vi "测试类型1can应答.vi"(0 "输入切换ID":u8, 1 "输出切换ID":u8, 3 "匹配CANID":u32 format="%x") -> (8 "成功？":bool)   [LabVIEW 2010]
uses:
  全局量/全局_配置.vi
panel:
  out "开始时间":dbl format="%#.0f"
  out "接收数据":u8[](array[numeric])
  out "超时?":bool
  in  "Baudrate":u32(ring)=1000 caption="K" items=["10"=10, "20"=20, "50"=50, "100"=100, "125"=125, "250"=250, "500"=500, "800"=800, "250"=1000]
  in  "CANPort":u16
  in  "ReadTimeOut":u32=3000 caption="ms"
  in  "Synchronization":i32(ring)=1 items=["Synchronization"=1, "Asynchronization"=0]
  out "Error out":errorcluster {"code" format="%.0x"}
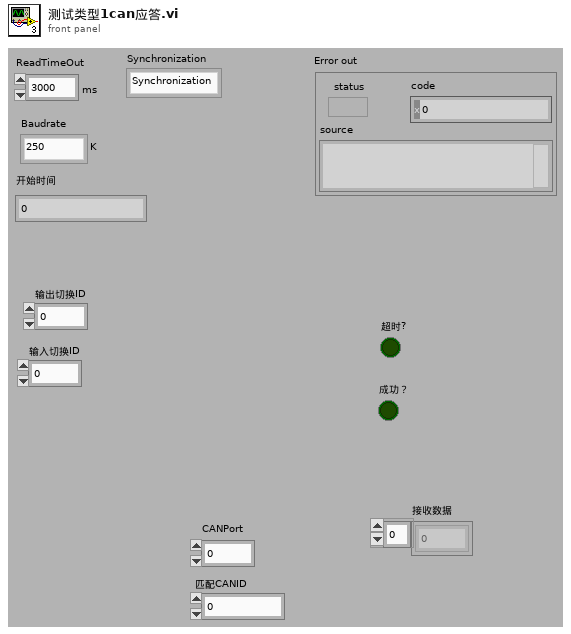
[diagram p1: front panel]
types:
  T1 = cluster{"Internal":u32, "InternalHigh":u32, "Offset":u32, "OffsetHigh":u32, "hEvent":u32}
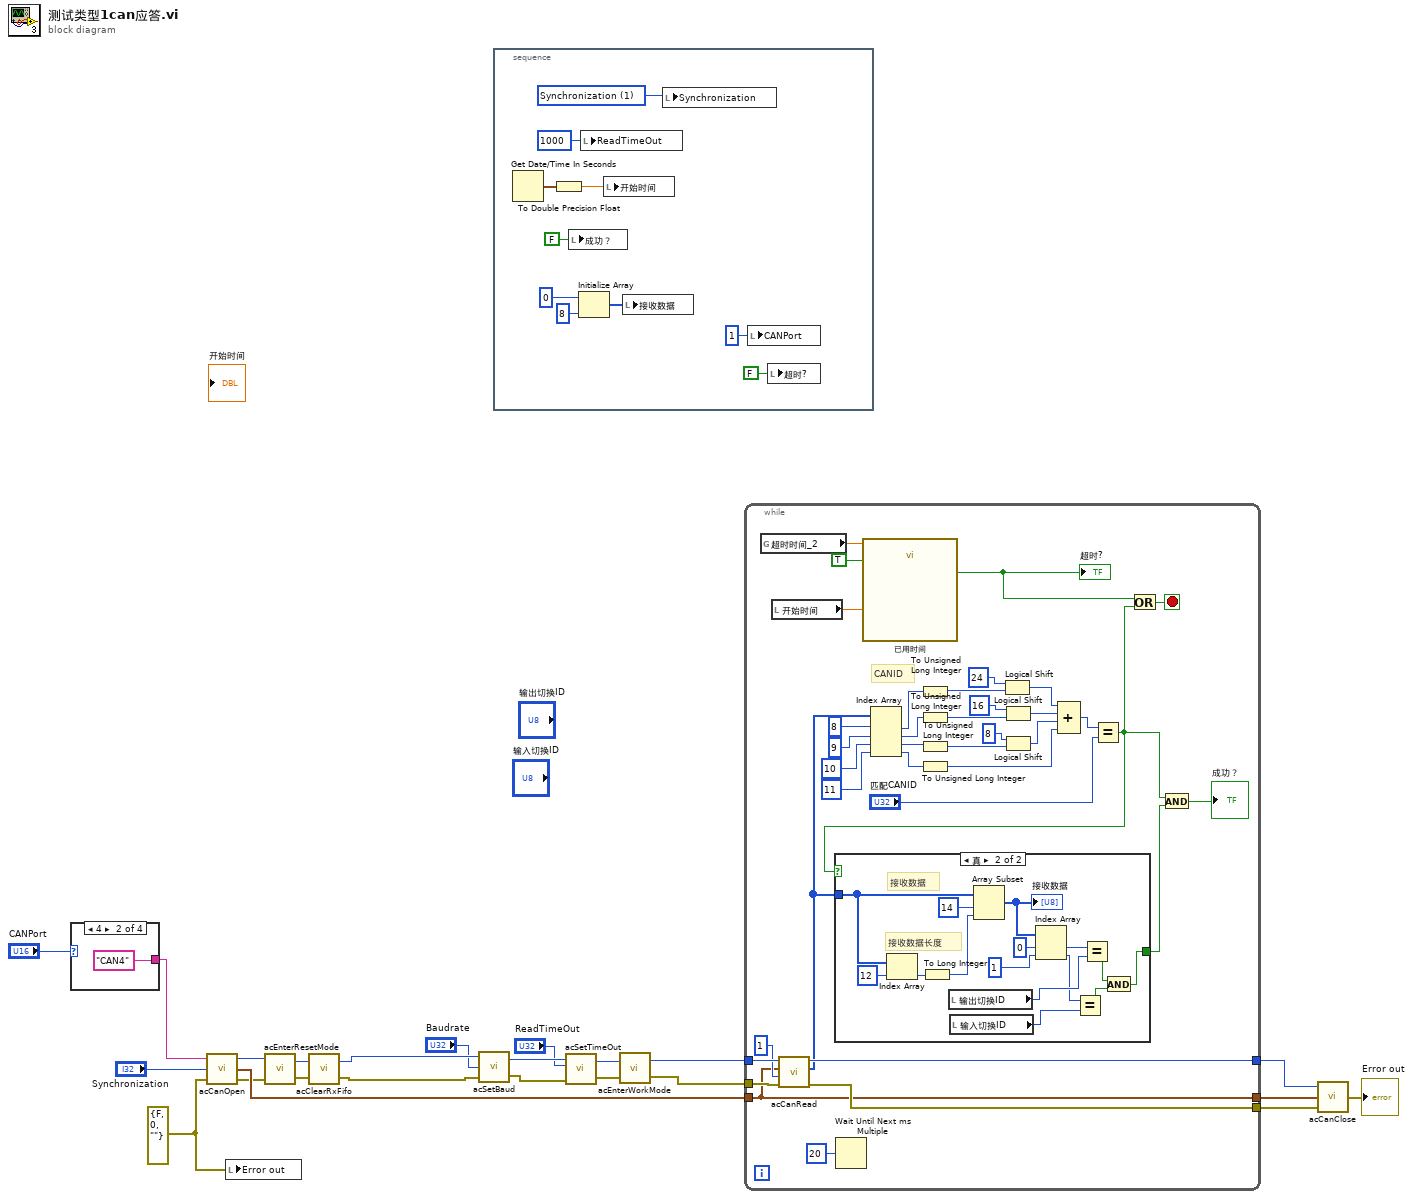
[diagram p0: block diagram]
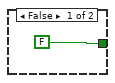
[diagram p2: hidden frame]
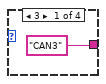
[diagram p3: hidden frame]
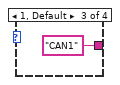
[diagram p4: hidden frame]
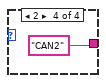
[diagram p5: hidden frame]
diagram:
  w17 = errorcluster {"status"=FALSE, "code"=0, "source"=""} ("Error in")
  n1 = case shown="4" "CANPort" {
    tunnel: ["CAN3" "CAN4" "CAN1" "CAN2"] -> w2
    frame 3 {
    }
    frame 4 {
    }
    frame 1, Default {
    }
    frame 2 {
    }
  }
  n2 = call "acCanOpen.vi"("Error in"=w17, "Synchronization"="Synchronization", "CANPort"=w2) -> ("Error out"=w18:errorcluster, "Overlapped"=w21:T1, "Handle"=w19:u32)
  n3 = local write "Error out"(w17) -> ()
  n4 = call "acEnterResetMode.vi"("Error in"=w18, "Handle  in"=w19) -> ("Error out"=w12:errorcluster, "Handle out"=w11:u32)
  n5 = call "acClearRxFifo.vi"("Error in"=w12, "Handle  in"=w11) -> ("Error out"=w9:errorcluster, "Handle out"=w10:u32)
  n6 = call "acSetBaud.vi"("Error in"=w9, "Baudrate"="Baudrate", "Handle  in"=w10) -> ("Error out"=w14:errorcluster, "Handle out"=w15:u32)
  n7 = stacked-sequence {
    frame #0 {
      w35 = 1 items=["Synchronization"=1, "Asynchronization"=0] ("Synchronization")
      n8 = Get Date/Time In Seconds() -> (seconds since 1Jan1904=w31:timestamp)
      n9 = To Double Precision Float(number=w31) -> (double precision float=w30:dbl)
      n10 = local write "成功？"(FALSE ("成功？")) -> ()
      n11 = Initialize Array(u8 0, 8 ("维数大小")) -> (w32:u8[])
      n12 = local write "ReadTimeOut"(u32 1000 ("ReadTimeOut")) -> ()
      n13 = local write "开始时间"(w30) -> ()
      n14 = local write "接收数据"(w32) -> ()
      n15 = local write "Synchronization"(w35) -> ()
      n16 = local write "CANPort"(u16 1 ("CANPort")) -> ()
      n17 = local write "超时?"(FALSE ("超时?")) -> ()
    }
  }
  n18 = call "acSetTimeOut.vi"("Error in"=w14, "Read TimeOut"="ReadTimeOut", "Handle  in"=w15) -> ("Error out"=w7:errorcluster, "Handle out"=w8:u32)  [unwired: 1 in]
  n19 = call "acEnterWorkMode.vi"("Error in"=w7, "Handle  in"=w8) -> ("Error out"=w5:errorcluster, "Handle out"=w6:u32)
  n20 = while {
    tunnel: [w73] -> w22
    tunnel: w21 -> [w68]
    tunnel: [w72] -> w20
    tunnel: w6 -> [w71]
    tunnel: w5 -> [w70]
    tunnel: [w68] -> w1
    stop <- w64 stop-if-true
    # "CANID"
    n21 = global read "全局_配置.vi" "超时时间_2"() -> (w66:dbl)
    n22 = local read "开始时间"() -> (w65:dbl)
    n23 = call "acCanRead.vi"("Error in"=w70, "ReadCount"=u32 1 ("接收CAN帧数 2"), "Overlapped"=w68, "Handle  in"=w71) -> ("Error out"=w72:errorcluster, "MSG"=w42:u8[], "Handle out"=w73:u32)  [unwired: 1 out]
    n24 = Wait Until Next ms Multiple(millisecond multiple=u32 20 ("毫秒倍数")) -> ()  [unwired: 1 out]
    n25 = call "已用时间"("Time Target (s)"=w66, "Reset"=TRUE, "Set Start Time (s)"=w65) -> ("Time has Elapsed"=w38:bool)  [unwired: 9 in, 7 out]
    "超时?" <- w38
    n26 = Index Array(array=w42, index #1=8 ("索引"), index #2=9 ("索引"), index #3=10 ("索引"), index #4=11 ("索引")) -> (element #1=w49:u8, element #2=w48:u8, element #3=w45:u8, element #4=w44:u8)
    n27 = To Unsigned Long Integer(number=w49) -> (unsigned 32bit integer=w50:u32)
    n28 = To Unsigned Long Integer(number=w48) -> (unsigned 32bit integer=w47:u32)
    n29 = To Unsigned Long Integer(number=w45) -> (unsigned 32bit integer=w46:u32)
    n30 = To Unsigned Long Integer(number=w44) -> (unsigned 32bit integer=w43:u32)
    n31 = Logical Shift(y=i8 24, x=w50) -> (x << y=w54:u32)
    n32 = Logical Shift(y=i8 16, x=w47) -> (x << y=w55:u32)
    n33 = Logical Shift(y=i8 8, x=w46) -> (x << y=w53:u32)
    n34 = Compound Arithmetic op=ADD(w54, w55, w53, w43) -> (w52:u32)
    n35 = Equal?(x=w52, y="匹配CANID") -> (x = y?=w41:bool)
    n36 = case shown="真" w41 {
      tunnel: w42 -> [_ w85]
      tunnel: [FALSE w75] -> w40
      frame False {
      }
      frame True {
        # "接收数据"
        # "接收数据长度"
        n37 = Index Array(array=w85, index=12 ("索引")) -> (element=w87:u8)
        n38 = To Long Integer(number=w87) -> (32bit integer=w86:i32)
        n39 = local read "输出切换ID"() -> (w80:u8)
        n40 = local read "输入切换ID"() -> (w78:u8)
        n41 = Array Subset(array=w85, index=14 ("索引"), length=w86) -> (w84:u8[])
        "接收数据" <- w84
        n42 = Index Array(array=w84, index #1=0 ("索引"), index #2=1 ("索引")) -> (element #1=w82:u8, element #2=w79:u8)
        n43 = Equal?(x=w79, y=w78) -> (x = y?=w76:bool)
        n44 = Equal?(x=w82, y=w80) -> (x = y?=w77:bool)
        n45 = And(x=w77, y=w76) -> (x .and. y?=w75:bool)
      }
    }
    n46 = Or(x=w38, y=w41) -> (x .or. y?=w64:bool)
    n47 = And(x=w41, y=w40) -> (x .and. y?=→"成功？":bool)
  }
  n48 = call "acCanClose.vi"("Error in"=w20, "Overlapped"=w1, "Handle  in"=w22) -> ("Error out"=→"Error out":errorcluster)
